vi "logic.vi"(9 "Elapsed time in current state":dbl format="%.2f", 11 "Plant State in":T1=1 items=["OFF"]) -> (2 "Rule name":string, 3 "Plant State out":T1=1 items=["OFF"])   [LabVIEW 2012]
uses:
  Plant state.ctl
  logic buffer cmd.ctl
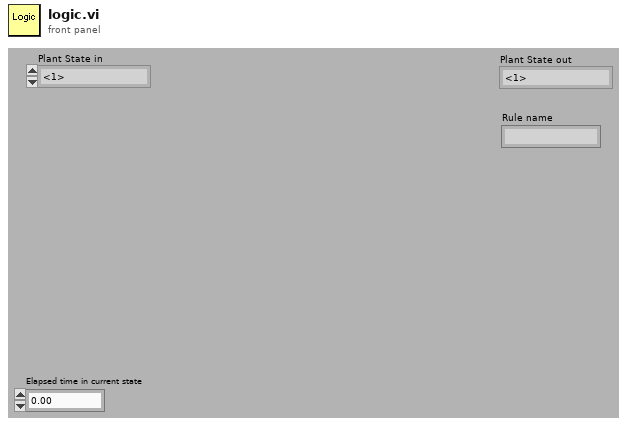
[diagram p1: front panel]
types:
  T1 = typedef "Plant state.ctl" = u16
  T2 = typedef "logic buffer cmd.ctl" = enum16{"read", "write ouput settings", "write rules", "write setpoints", "write output descriptions", "write all", "calculate setpoints", "save", "open", "Load all setpoint code", "Load one setpoint code", "Configure one setpoint code"}
  T3 = typedef "variable setpoint.ctl" = cluster{"name":string, "unit":string, "value":dbl, "Type":enum16{"Constant", "Variable"}, "variable":cluster{"selected sensors":i32[], "selected set points":i32[], "VI":path, "Data average interval":T4, "code ref":T5}}
  T4 = typedef "data ave interval.ctl" = dbl
  T5 = typedef "type specifier for control code.ctl" = refnum<vi>
  T6 = typedef "rules.ctl" = T7[]
  T7 = typedef "State rules.ctl" = cluster{"state rules":T8[], "State name":string}
  T8 = typedef "rule.ctl" = cluster{"next state":u16, "conditions":T9[], "number of conditions":u8, "Rule name":string}
  T9 = typedef "condition.ctl" = cluster{"> or <":T10, "set point":i32, "sensors and variables":i32, "Data average interval":dbl}
  T10 = typedef "greater or less.ctl" = bool
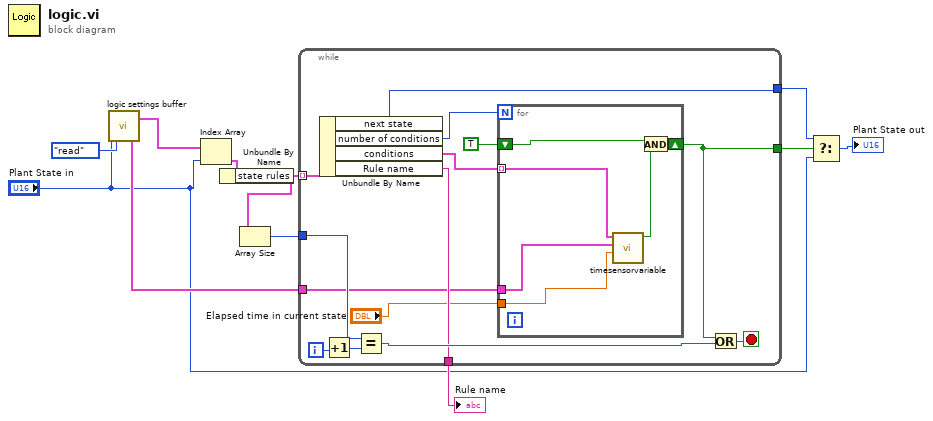
[diagram p0: block diagram]
diagram:
  n1 = call "logic settings buffer.vi"("Plant  state"="Plant State in", "command"=logic_buffer_cmd."read") -> ("Set Points out"=w3:T3[], "Rules out"=w4:T6)  [unwired: 10 in, 6 out]
  n2 = Index Array(array=w4, index="Plant State in") -> (element=w11:T7)
  n3 = Unbundle By Name(w11) -> ("state rules"=w10:T8[])
  n4 = Array Size(array=w10) -> (size(s)=w9:i32)
  n5 = while {
    tunnel: w10 -> [w25] mode=indexing
    tunnel: w9 -> [w21]
    tunnel: [w16] -> w8
    tunnel: [w15] -> w7
    tunnel: [w14] -> w6
    tunnel: w3 -> [w13]
    i -> [w20]
    stop <- w17 stop-if-true
    n6 = Unbundle By Name(w25) -> ("next state"=w15:u16, "number of conditions"=w24:u8, "conditions"=w23:T9[], "Rule name"=w14:string)
    n7 = Increment(x=w20) -> (x+1=w19:i32)
    n8 = Equal?(x=w21, y=w19) -> (x = y?=w18:bool)
    n9 = for {
      N: w24 -> [_]
      tunnel: w23 -> [w27] mode=indexing
      shift-right: [w31] -> w16
      shift-left: TRUE -> [w30]
      tunnel: w13 -> [w29]
      tunnel: "Elapsed time in current state" -> [w28]
      n10 = call "timesensorvariable.vi"("Elapsed time in current state"=w28, "S P & V definitions"=w29, "condition"=w27) -> ("exit"=w26:bool)  [unwired: 8 in]
      n11 = And(x=w30, y=w26) -> (x .and. y?=w31:bool)
    }
    n12 = Or(x=w16, y=w18) -> (x .or. y?=w17:bool)
  }
  "Rule name" <- w6
  n13 = Select(t=w7, s=w8, f="Plant State in") -> (s? t:f=→"Plant State out":T1)
